vi "Compute Distance.vi"(8 "Y Image Resolution":i32, 9 "X Image Resolution":i32, 10 "Bounding Box":T1, 11 "Camera Type":enum16{"206", "1011"}(ring)) -> (0 "Distance (m)":dbl, 1 "Target Center (Camera)":cluster{"X":dbl, "Y":dbl}, 2 "Target Center (-1 to 1)":cluster{"X":dbl, "Y":dbl}, 3 "Distance (ft)":dbl)   [LabVIEW 2011]
doc: "Using the camera lens information and the real world width of the target, determine the distance to the target."
panel:
  in  "Camera view angle":dbl[](array[numeric])=[48.0, 43.5]
  # "Axis 206\nAxis M1011"
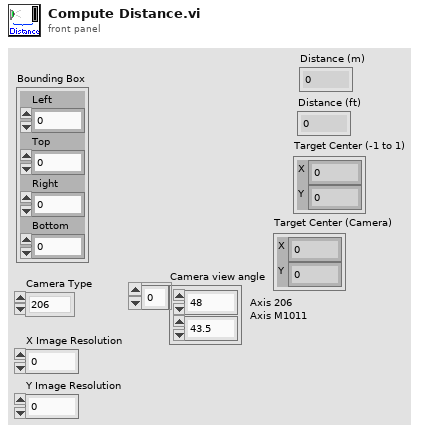
[diagram p1: front panel]
types:
  T1 = cluster{"Left":dbl, "Top":dbl, "Right":dbl, "Bottom":dbl}
  T2 = cluster{"X Image Resolution":i32, "Y Image Resolution":i32}
  T3 = cluster{"X Image Resolution":dbl, "Y Image Resolution":dbl}
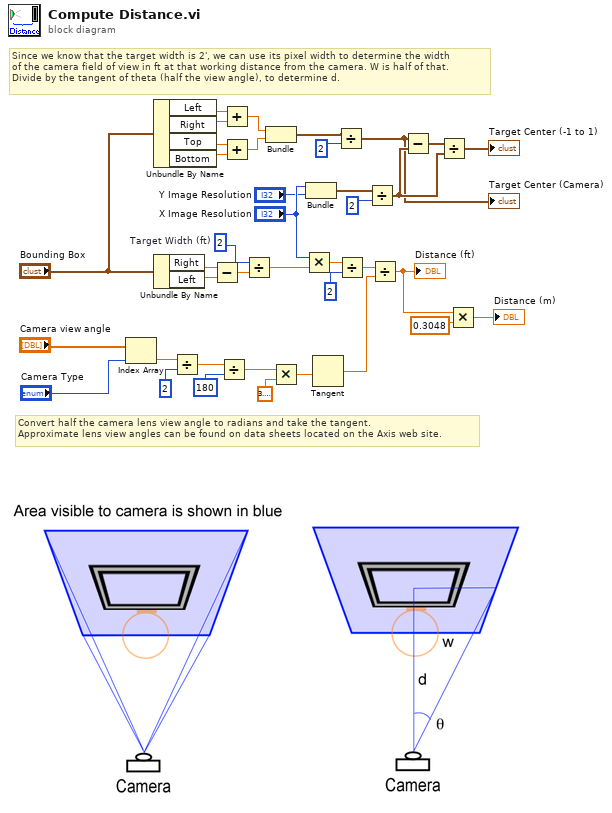
[diagram p0: block diagram]
diagram:
  w21 = 2  # Target Width (ft)
  # "Convert half the camera lens view angle to radians and take the tangent.\nApproximate lens view angles can be found on data sheets located on the Axis web site."
  # "Since we know that the target width is 2', we can use its pixel width to determine the width\nof the camera field of view in ft at that working distance from the camera. W is half of that.\nDivide by the tangent of theta (half the view angle), to determine d."
  n1 = Index Array(array="Camera view angle", index="Camera Type") -> (element=w34:dbl)
  n2 = Unbundle By Name("Bounding Box") -> ("Left"=w16:dbl, "Right"=w17:dbl, "Top"=w19:dbl, "Bottom"=w18:dbl)
  n3 = Unbundle By Name("Bounding Box") -> ("Right"=w25:dbl, "Left"=w24:dbl)
  n4 = Divide(x=w34, y=2) -> (x/y=w31:dbl)
  n5 = Subtract(x=w25, y=w24) -> (x-y=w23:dbl)
  n6 = Divide(x=w31, y=180) -> (x/y=w30:dbl)
  n7 = Add(x=w16, y=w17) -> (x+y=w14:dbl)
  n8 = Add(x=w19, y=w18) -> (x+y=w13:dbl)
  n9 = Divide(x=w21, y=w23) -> (x/y=w22:dbl)
  n10 = Bundle(w14, w13) -> (w8:cluster{dbl, dbl})  [unwired: 1 in]
  n11 = Multiply(x=w30, y=3.141592653589793) -> (x*y=w32:dbl)
  n12 = Multiply(x="X Image Resolution", y=w22) -> (x*y=w26:dbl)
  n13 = Bundle("X Image Resolution"="X Image Resolution", "Y Image Resolution"="Y Image Resolution") -> (w10:T2)  [unwired: 1 in]
  n14 = Tangent(1:w32) -> (0:w38:dbl)
  n15 = Divide(x=w8, y=2) -> (x/y=w4:cluster{dbl, dbl})
  "Target Center (Camera)" <- w4
  n16 = Divide(x=w26, y=2) -> (x/y=w28:dbl)
  n17 = Divide(x=w10, y=2) -> (x/y=w6:T3)
  n18 = Divide(x=w28, y=w38) -> (x/y=w3:dbl)
  "Distance (ft)" <- w3
  n19 = Subtract(x=w4, y=w6) -> (x-y=w7:cluster{dbl, dbl})
  n20 = Divide(x=w7, y=w6) -> (x/y=→"Target Center (-1 to 1)":cluster{dbl, dbl})
  n21 = Multiply(x=w3, y=0.3048) -> (x*y=→"Distance (m)":dbl)
